vi "PH_gentec_M-Link.set Autorange.vi"(0 "i ref in":refnum<vi>, 2 "VISA resource in":refnum<visa-resource-name>, 5 "error in":errorcluster) -> (11 "Timeout":bool, 13 "Data read":string[](array[string]), 14 "i ref out":refnum<vi>, 16 "VISA resource out":refnum<visa-resource-name>, 17 "Error":bool, 18 "Failure":bool, 19 "error out":errorcluster)   [LabVIEW 2014, in "PH_gentec_M-Link.lvlib"]
doc: "This VI writes wanted Settings to the Device and checks the result."
uses:
  PH_gentec_M-Link.lvlib
  instr.lib/Gentec-M-Link/Driver/Type Defs/gentec-M-Link.Range Queries.ctl
  instr.lib/Gentec-M-Link/gentec-M-Link - Driver.lvlib
  PH_Basics/PH_Powermeter_BaseClass/PH_Powermeter_BaseClass.lvlib
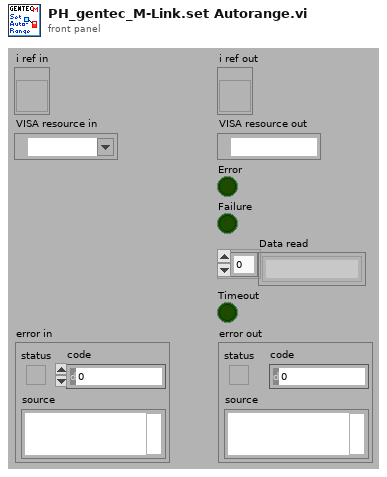
[diagram p1: front panel]
types:
  T1 = typedef "PH_gentec_M-Link.lvlib/PH_gentec_M-Link.i attribute.ctl" = cluster{"GUI References":cluster{"Wanted Head Settings":refnum<vi>, "Current Head Settings":refnum<vi>, "Set Auto Range":refnum<vi>, "Trigger Polarity":refnum<vi>, "Trigger Source":refnum<vi>, "Waveform Averages":refnum<vi>, "Continuous":refnum<vi>, "get one Value":refnum<vi>}, "Wanted Head Settings":T2, "Current Head Settings":T2}
  T2 = typedef "PH_gentec_M-Link.lvlib/PH_gentec_M-Link.Head Settings.ctl" = cluster{"Measurement Mode":T3, "Enable Anticipation":bool, "Set Auto Range":bool, "Block Signal":bool, "Set Head Attenuator":bool, "Enable SSE":bool, "Trigger Polarity":T4, "Trigger Source":T5, "Waveform Averages":T6, "Set Zero":i32, "Current":i32, "Start Data Flow":bool}
  T3 = typedef "gentec-M-Link - Driver.lvlib/gentec-M-Link.Measurement Mode.ctl" = u16
  T4 = typedef "gentec-M-Link - Driver.lvlib/gentec-M-Link.Trigger Polarity.ctl" = u16
  T5 = typedef "gentec-M-Link - Driver.lvlib/gentec-M-Link.Trigger Source.ctl" = u16
  T6 = typedef "gentec-M-Link - Driver.lvlib/gentec-M-Link.Waveform Averages.ctl" = u16
  T7 = typedef "gentec-M-Link - Driver.lvlib/gentec-M-Link.Range Queries.ctl" = string
  T8 = typedef "gentec-M-Link - Driver.lvlib/gentec-M-Link.Range.ctl" = u16
  T9 = typedef "PH_Powermeter_BaseClass.lvlib/PH_Powermeter_BaseClass.i attribute.ctl" = cluster{"GUI References":T10, "Connection":T11, "Head Attributes":T13, "VISA resource":refnum<visa-resource-name>, "Energy":T14, "Service ID Energy":i32, "Wanted Settings":T15, "Current Settings":T15}
  T10 = typedef "PH_Powermeter_BaseClass.lvlib/PH_Powermeter_BaseClass.GUI Refs.ctl" = cluster{"Head Attributes":refnum<vi>, "Energy":refnum<vi>, "Connection":refnum<vi>, "VISA Resource":refnum<vi>, "Scaling Factor":refnum<vi>, "Range":refnum<vi>, "Wavelength":refnum<vi>, "Trigger Level":refnum<vi>, "Wanted Settings":refnum<vi>, "Current Settings":refnum<vi>}
  T11 = typedef "PH_Powermeter_BaseClass.lvlib/PH_Powermeter_BaseClass.Connection.ctl" = cluster{"failed checks":i8, "Timeout":bool, "Data read":string, "Failure":bool, "Error":bool, "State":T12}
  T12 = typedef "PH_Powermeter_BaseClass.lvlib/PH_Powermeter_BaseClass.State.ctl" = enum32{"off", "operating", "opened", "checked", "connected", "Sets to change", "running"}
  T13 = typedef "PH_Powermeter_BaseClass.lvlib/PH_Powermeter_BaseClass.Head Attributes.ctl" = cluster{"Instrument Type":string, "Head Version":string, "Head Name":string, "Serial Number":string, "Firmware":string, "Sensor Type":string, "MinimumRange":u32, "Maximum Range":u32, "Min Wavelength":i32, "Max Wavelength":i32}
  T14 = typedef "PH_Powermeter_BaseClass.lvlib/PH_Powermeter_BaseClass.Energy.ctl" = cluster{"current Value":dbl, "unscaled":dbl, "Scaling Factor":dbl}
  T15 = typedef "PH_Powermeter_BaseClass.lvlib/PH_gentec_BaseClass.Head Settings.ctl" = cluster{"Trigger Level":dbl, "Wavelength":u32, "Range":u32}
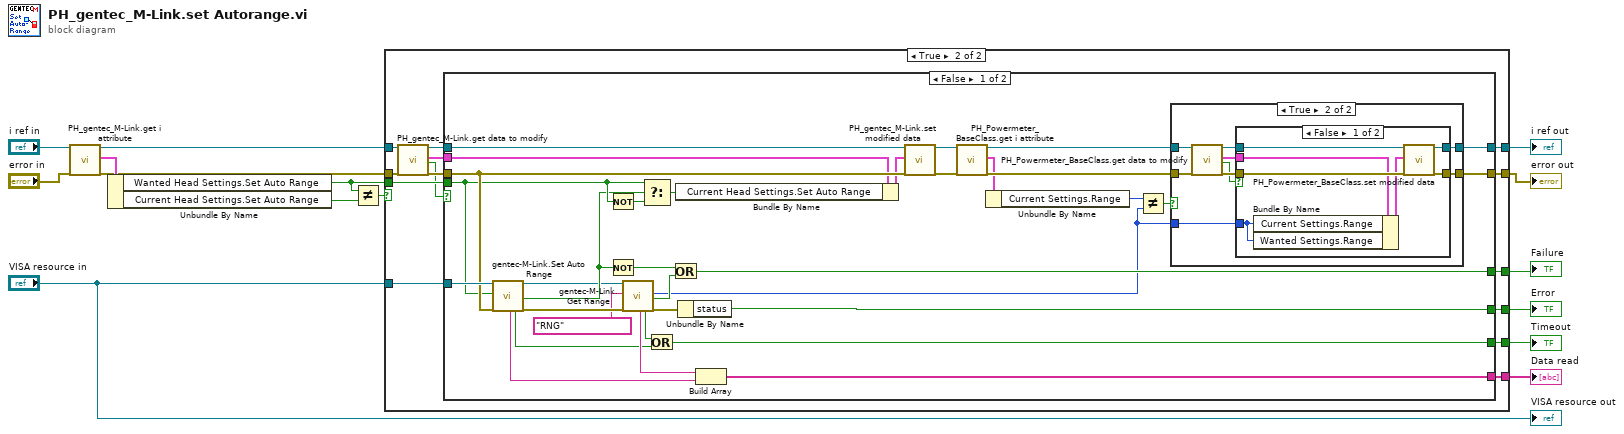
[diagram p0: block diagram]
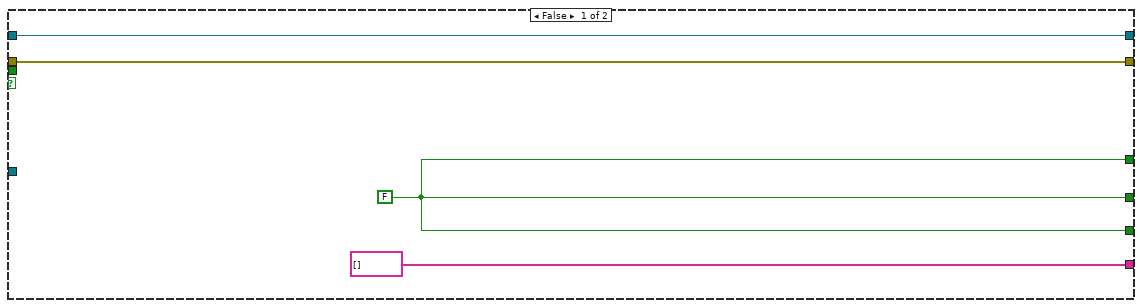
[diagram p2: hidden frame]
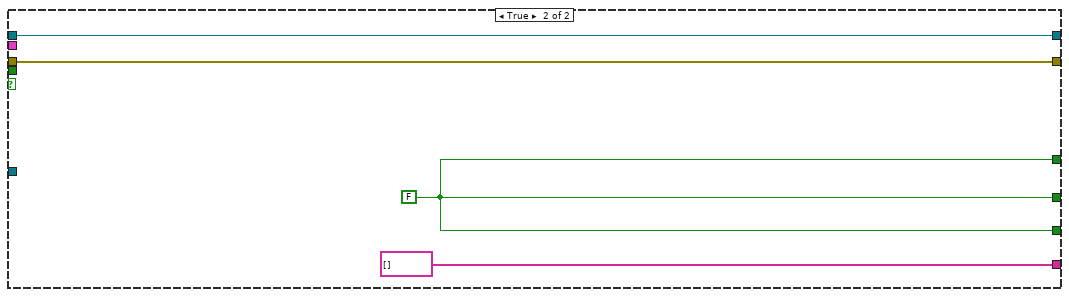
[diagram p5: hidden frame]
diagram:
  n1 = call "PH_gentec_M-Link.get i attribute.vi"("i ref in"="i ref in", "error in (no error)"="error in") -> ("i ref out"=w8:refnum<vi>, "i attribute"=w11:T1, "error out"=w10:errorcluster)  [unwired: 15 in]
  n2 = Unbundle By Name(w11) -> ("Wanted Head Settings.Set Auto Range"=w12:bool, "Current Head Settings.Set Auto Range"=w13:bool)
  n3 = Not Equal?(x=w12, y=w13) -> (x != y?=w1:bool)
  n4 = case shown="True" w1 {
    tunnel: [w18 w33] -> w15
    tunnel: [w19 w32] -> w14
    tunnel: w12 -> [_ w31]
    tunnel: w10 -> [w18 w26]
    tunnel: w8 -> [w19 w25]
    tunnel: "VISA resource in" -> [_ w24]
    tunnel: [string[] [] w23] -> w5
    tunnel: [w17 w22] -> w4
    tunnel: [w17 w21] -> w3
    tunnel: [w17 w20] -> w2
    frame False {
      w17 = FALSE
    }
    frame True {
      n5 = call "PH_gentec_M-Link.get data to modify.vi"("i ref in"=w25, "error in (no error)"=w26) -> ("i ref out"=w29:refnum<vi>, "i attribute"=w28:T1, "timed out"=w27:bool, "error out"=w30:errorcluster)  [unwired: 14 in]
      n6 = case shown="False" w27 {
        tunnel: w24 -> [w65 _]
        tunnel: [w36 w90] -> w32
        tunnel: [w35 w89] -> w33
        tunnel: w30 -> [w64 w89]
        tunnel: w29 -> [w66 w90]
        tunnel: w28 -> [w47 _]
        tunnel: w31 -> [w62 _]
        tunnel: [w49 string[] []] -> w23
        tunnel: [w46 w87] -> w22
        tunnel: [w45 w87] -> w21
        tunnel: [w44 w87] -> w20
        frame False {
          n7 = call "gentec-M-Link.Set Auto Range.vi"("VISA resource In"=w65, "Auto Range"=w62, "error in (no error)"=w64) -> ("Data Read"=w54:string, "Read Timeout"=w51:bool, "VISA resource Out"=w57:refnum<visa-resource-name>, "Success"=w61:bool, "error out"=w59:errorcluster)  [unwired: 12 in]
          n8 = Not(x=w62) -> (.not. x?=w60:bool)
          n9 = Not(x=w61) -> (.not. x?=w52:bool)
          n10 = call "gentec-M-Link.Get Range.vi"("VISA resource In"=w57, "Range Queries"=T7 "RNG", "error in (no error)"=w59) -> ("Data Read"=w55:string, "Read Timeout"=w50:bool, "Range"=w34:T8, "Error"=w53:bool, "error out"=w58:errorcluster)  [unwired: 11 in, 1 out]
          n11 = Select(t=w62, s=w61, f=w60) -> (s? t:f=w48:bool)
          n12 = Or(x=w50, y=w51) -> (x .or. y?=w46:bool)
          n13 = Or(x=w52, y=w53) -> (x .or. y?=w44:bool)
          n14 = Bundle By Name(cluster=w47, "Current Head Settings.Set Auto Range"=w48) -> (w63:T1)
          n15 = Unbundle By Name(w58) -> ("status"=w45:bool)
          n16 = Build Array(w55, w54) -> (w49:string[])
          n17 = call "PH_gentec_M-Link.set modified data.vi"("i ref in"=w66, "i attribute"=w63, "error in (no error)"=w64) -> ("i ref out"=w38:refnum<vi>, "error out"=w37:errorcluster)  [unwired: 15 in]
          n18 = call "PH_Powermeter_BaseClass.get i attribute.vi"("i ref in"=w38, "error in (no error)"=w37) -> ("i ref out"=w42:refnum<vi>, "i attribute"=w40:T9, "error out"=w41:errorcluster)  [unwired: 15 in]
          n19 = Unbundle By Name(w40) -> ("Current Settings.Range"=w39:u32)
          n20 = Not Equal?(x=w39, y=w34) -> (x != y?=w43:bool)
          n21 = case shown="True" w43 {
            tunnel: [w67 w77] -> w35
            tunnel: [w68 w76] -> w36
            tunnel: w41 -> [w67 w71]
            tunnel: w42 -> [w68 w70]
            tunnel: w34 -> [_ w69]
            frame False {
            }
            frame True {
              n22 = call "PH_Powermeter_BaseClass.get data to modify.vi"("i ref in"=w70, "error in (no error)"=w71) -> ("i ref out"=w74:refnum<vi>, "i attribute"=w73:T9, "timed out"=w72:bool, "error out"=w75:errorcluster)  [unwired: 14 in]
              n23 = case shown="False" w72 {
                tunnel: [w81 w86] -> w76
                tunnel: [w80 w85] -> w77
                tunnel: w75 -> [w83 w85]
                tunnel: w74 -> [w84 w86]
                tunnel: w73 -> [w82 _]
                tunnel: w69 -> [w78 _]
                frame False {
                  n24 = Bundle By Name(cluster=w82, "Current Settings.Range"=w78, "Wanted Settings.Range"=w78) -> (w79:T9)
                  n25 = call "PH_Powermeter_BaseClass.set modified data.vi"("i ref in"=w84, "i attribute"=w79, "error in (no error)"=w83) -> ("i ref out"=w81:refnum<vi>, "error out"=w80:errorcluster)  [unwired: 15 in]
                }
                frame True {
                }
              }
            }
          }
        }
        frame True {
          w87 = FALSE
        }
      }
    }
  }
  "error out" <- w15
  "i ref out" <- w14
  "Data read" <- w5
  "Timeout" <- w4
  "Error" <- w3
  "Failure" <- w2
  "VISA resource out" <- "VISA resource in"
